vi "Host_Panel.vi"() -> ()   [LabVIEW 2024]
uses:
  TensionChart.ctl
panel:
  out "Tension Telemetry Error":errorcluster
  out "TensionChart 14":T1 caption="1"
  out "TensionChart 13":T1 caption="1"
  out "TensionChart 12":T1 caption="1"
  out "TensionChart 11":T1 caption="1"
  out "TensionChart 10":T1 caption="1"
  out "TensionChart 9":T1 caption="1"
  out "TensionChart 8":T1 caption="1"
  out "TensionChart 7":T1 caption="1"
  out "TensionChart 6":T1 caption="1"
  out "TensionChart 5":T1 caption="1"
  out "TensionChart 4":T1 caption="1"
  out "TensionChart 3":T1 caption="1"
  out "TensionChart 2":T1 caption="1"
  out "TensionChart 1":T1 caption="1"
  in  "Stop Host":bool
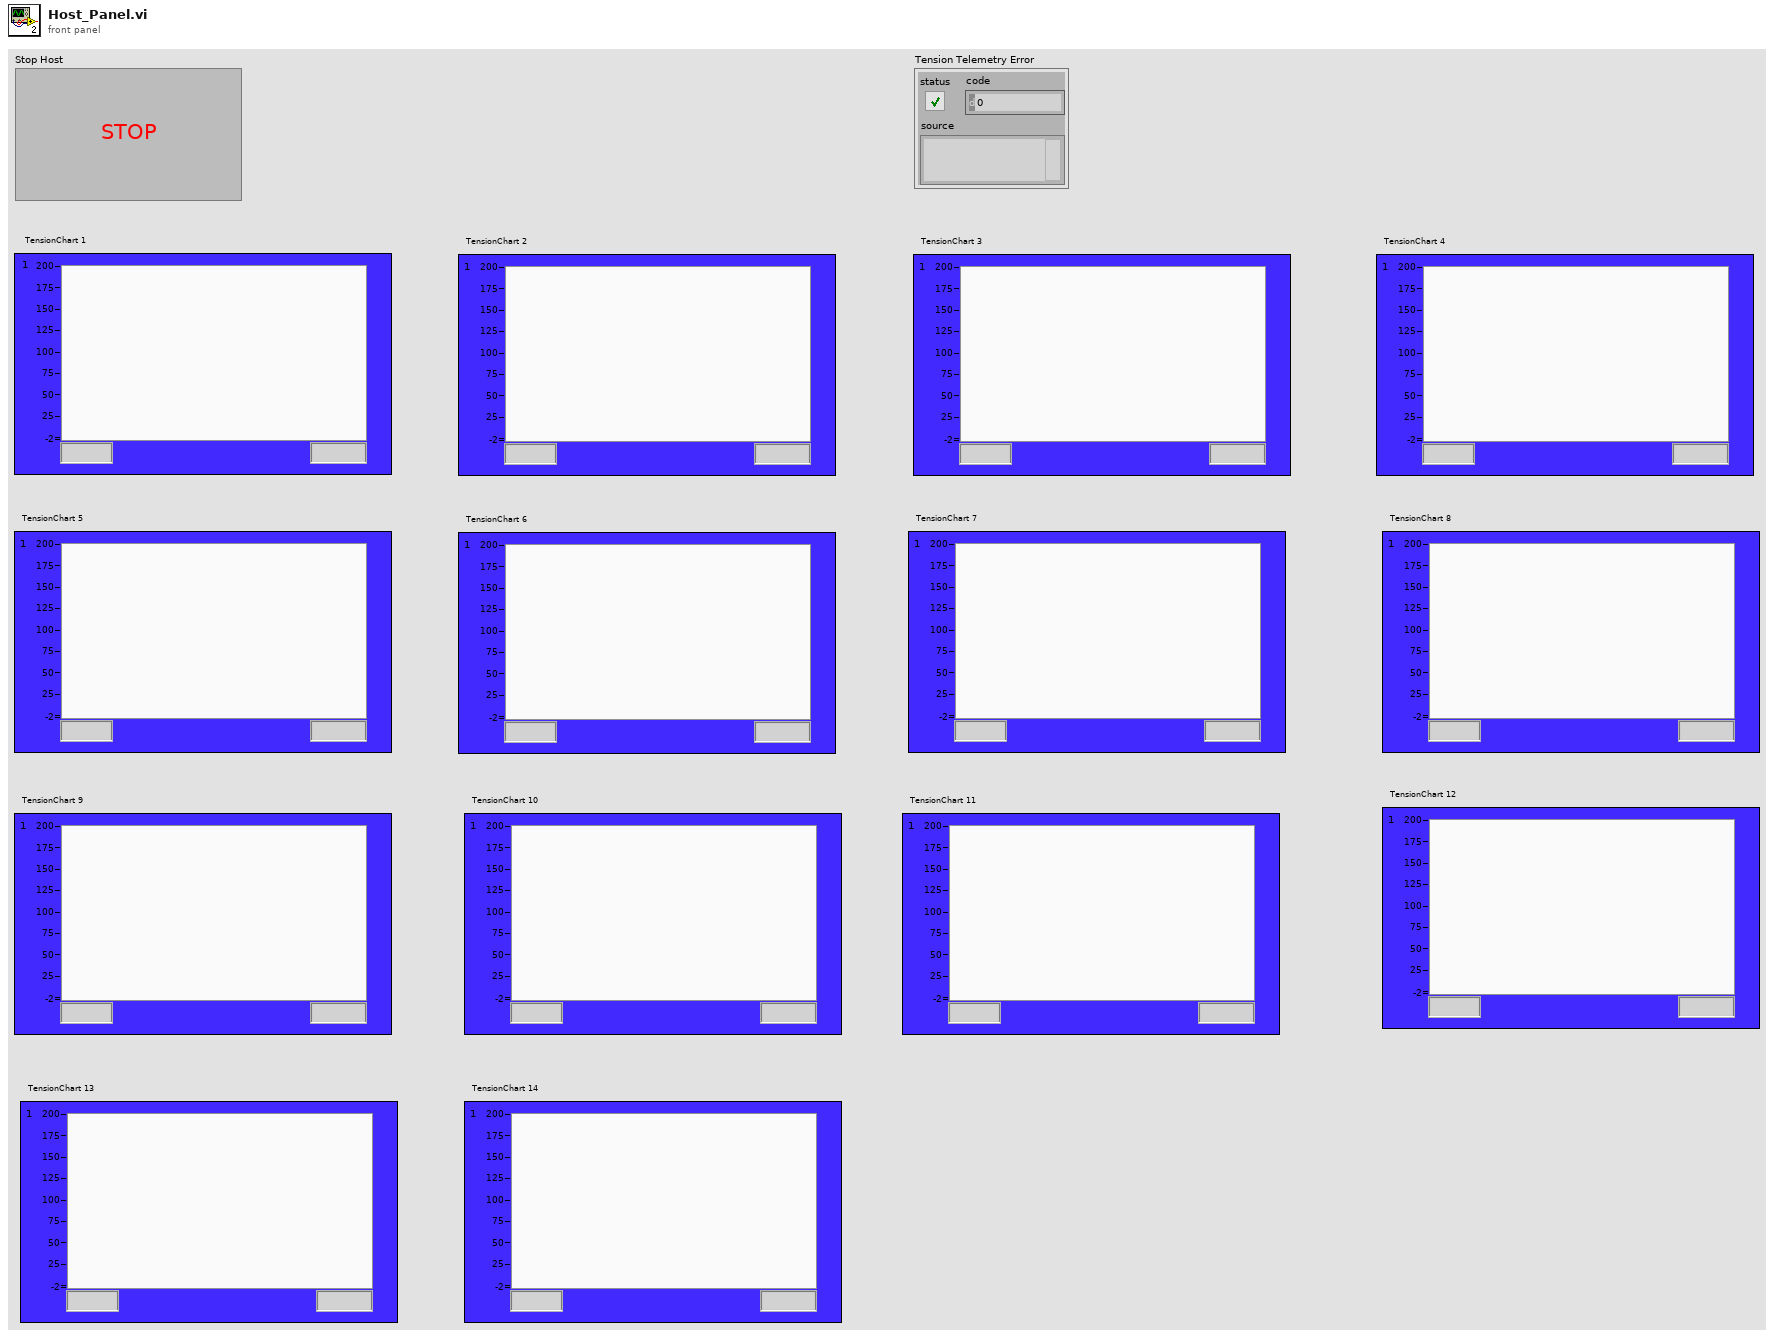
[diagram p1: front panel]
types:
  T1 = typedef "TensionChart.ctl" = cluster{"[0]":dbl, "[1]":dbl}
  T2 = cluster{"curr_Tensions":dbl[], "goal_Tensions":dbl[]}
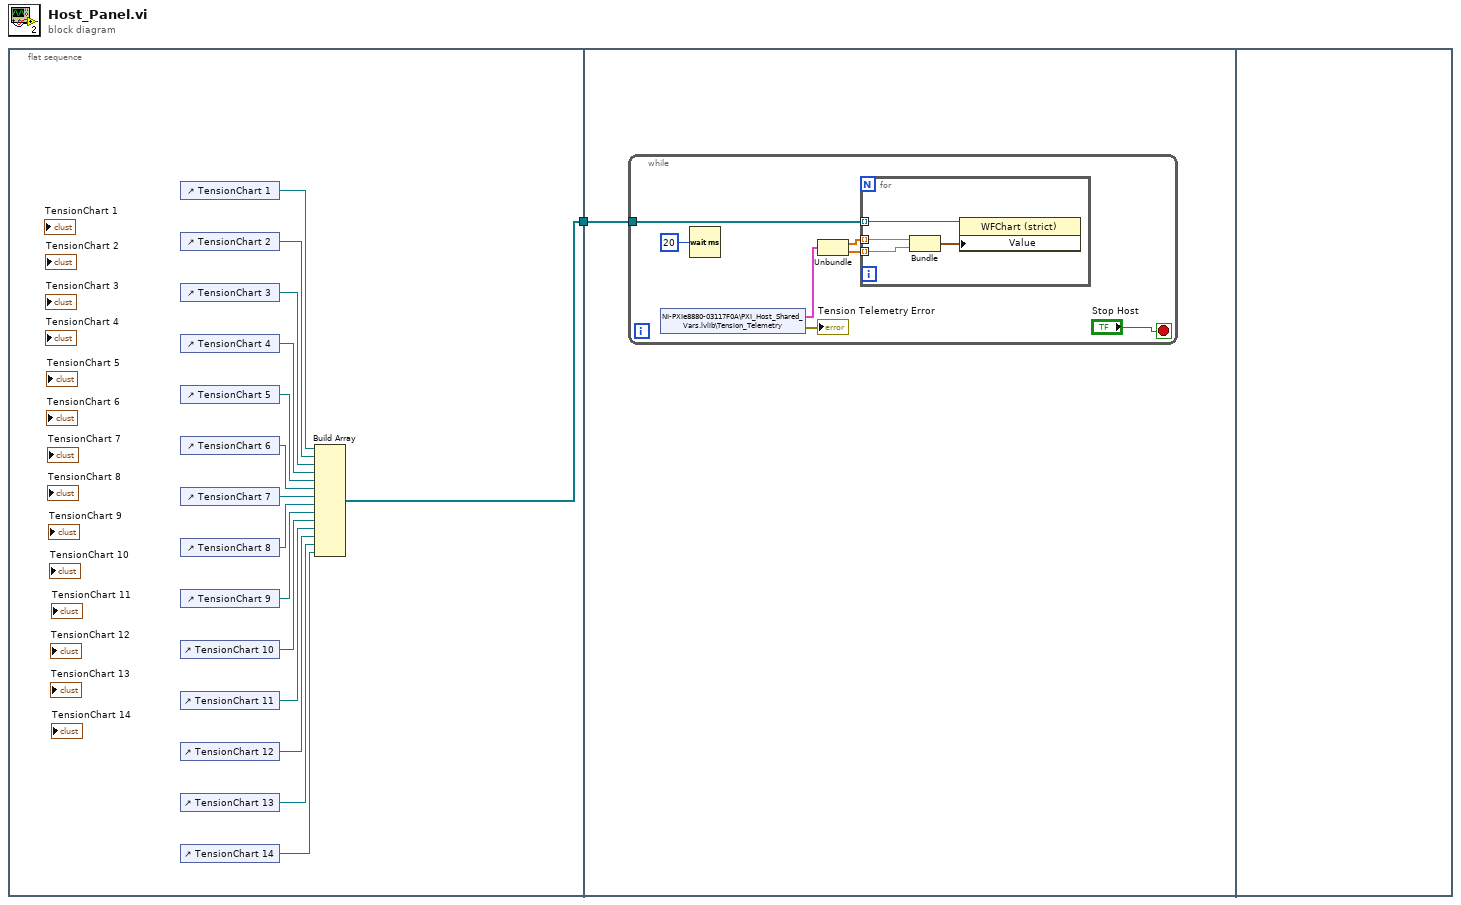
[diagram p0: block diagram]
diagram:
  n1 = flat-sequence {
    tunnel: [w2] -> w1
    tunnel: w1 -> [w17]
    frame #0 {
      n2 = control-ref of="TensionChart 1"() -> (w16:refnum<vi>)
      n3 = control-ref of="TensionChart 2"() -> (w15:refnum<vi>)
      n4 = control-ref of="TensionChart 3"() -> (w14:refnum<vi>)
      n5 = control-ref of="TensionChart 4"() -> (w13:refnum<vi>)
      n6 = control-ref of="TensionChart 5"() -> (w12:refnum<vi>)
      n7 = control-ref of="TensionChart 6"() -> (w11:refnum<vi>)
      n8 = control-ref of="TensionChart 7"() -> (w10:refnum<vi>)
      n9 = control-ref of="TensionChart 8"() -> (w9:refnum<vi>)
      n10 = control-ref of="TensionChart 9"() -> (w8:refnum<vi>)
      n11 = control-ref of="TensionChart 10"() -> (w7:refnum<vi>)
      n12 = control-ref of="TensionChart 11"() -> (w6:refnum<vi>)
      n13 = control-ref of="TensionChart 12"() -> (w5:refnum<vi>)
      n14 = control-ref of="TensionChart 13"() -> (w4:refnum<vi>)
      n15 = control-ref of="TensionChart 14"() -> (w3:refnum<vi>)
      n16 = Build Array(w16, w15, w14, w13, w12, w11, w10, w9, w8, w7, w6, w5, w4, w3) -> (w2:refnum<vi>[])
    }
    frame #1 {
      n17 = while {
        tunnel: w17 -> [w20]
        stop <- "Stop Host" stop-if-true
        n18 = shared-variable "NI-PXIe8880-03117F0A\\PXI_Host_Shared_Vars.lvlib\\Tension_Telemetry"() -> (w22:T2, error out=→"Tension Telemetry Error":errorcluster)  [unwired: 1 in]
        n19 = Wait (ms)(milliseconds to wait=u32 20) -> ()  [unwired: 1 out]
        n20 = Unbundle(w22) -> ("curr_Tensions"=w19:dbl[], "goal_Tensions"=w18:dbl[])
        n21 = for {
          tunnel: w20 -> [w26] mode=indexing
          tunnel: w19 -> [w28] mode=indexing
          tunnel: w18 -> [w27] mode=indexing
          n22 = Bundle("element"=w28, "element"=w27) -> (w25:cluster{"element":dbl, "element":dbl})  [unwired: 1 in]
          n23 = property class="WFChart (strict)"(reference=w26, "Value"=w25) -> ()  [unwired: 1 in, 2 out]
        }
      }
    }
    frame #2 {
    }
  }
